vi "Email_to_rcpt.vi"(3 "Email Addresses":string[](array[string])) -> (0 "rcpt to":string[](array[string]), 1 "To":string)   [LabVIEW 2010]
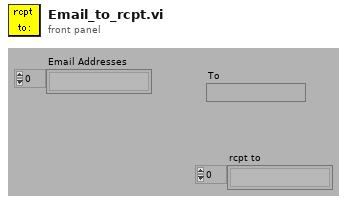
[diagram p1: front panel]
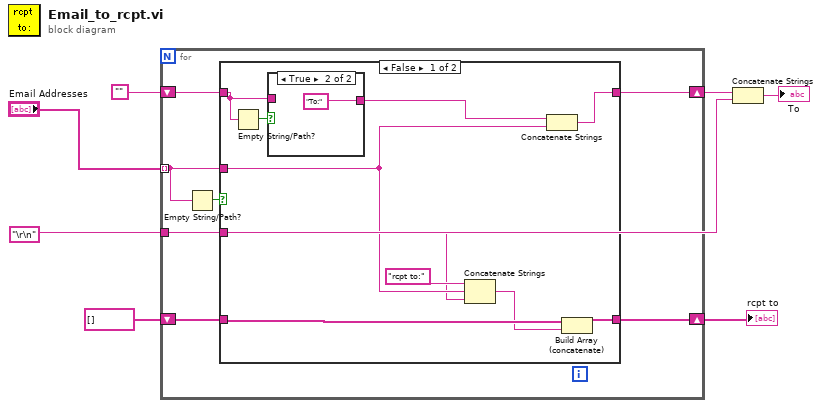
[diagram p0: block diagram]
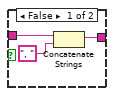
[diagram p2: hidden frame]
diagram:
  w2 = "\r\n"
  n1 = for {
    tunnel: "Email Addresses" -> [w10] mode=indexing
    tunnel: w2 -> [w12]
    shift-right: [w13] -> w3
    shift-left: "" -> [w14]
    shift-right: [w9] -> w5
    shift-left: string[] [] -> [w8]
    n2 = Empty String/Path?(string/path=w10) -> (empty?=w11:bool)
    n3 = case shown="False" w11 {
      tunnel: w10 -> [w23 _]
      tunnel: w14 -> [w15 w30]
      tunnel: [w22 w30] -> w13
      tunnel: w12 -> [w21 _]
      tunnel: [w19 w29] -> w9
      tunnel: w8 -> [w20 w29]
      frame False {
        n4 = Empty String/Path?(string/path=w15) -> (empty?=w17:bool)
        n5 = case shown="True" w17 {
          tunnel: [w27 "To:"] -> w16
          tunnel: w15 -> [w26 _]
          frame False {
            n6 = Concatenate Strings(w26, ", " ("Substring")) -> (w27:string)
          }
          frame True {
          }
        }
        n7 = Concatenate Strings("rcpt to:", w23, w21) -> (w18:string)
        n8 = Concatenate Strings(w16, w23) -> (w22:string)
        n9 = Build Array (concatenate)(w20, w18) -> (w19:string[])
      }
      frame True {
      }
    }
  }
  "rcpt to" <- w5
  n10 = Concatenate Strings(w3, w2) -> (→"To":string)
